vi "Initialize Serial Arm.vi"   [LabVIEW 2017, in "NI_Robotics_AnalyticKinematics.lvlib"]
doc: "Sets the properties of a serial robot arm and generates a representation of the arm. If you have access to a 6R, 5R, or SCARA arm, generate that type of arm. If you do not have access to an arm of those types, generate a generic arm. You must manually select the polymorphic instance to use."
uses:
  <vilib>/robotics/Kinematics/Analytical/NI_Robotics_AnalyticKinematics.lvlib
  <vilib>/robotics/Kinematics/Analytical/6R/Type 1/NI_Robotics_6R Type 1 Serial Arm Class.lvclass
  <vilib>/robotics/Kinematics/Robot/NI_Robotics_Serial Robot Arm.lvclass
  <vilib>/robotics/Kinematics/Analytical/SCARA/NI_Robotics_SCARA Serial Arm Class.lvclass
  <vilib>/robotics/Kinematics/Analytical/6R/Type 3/NI_Robotics_6R Type 3 Serial Arm Class.lvclass
  <vilib>/robotics/Kinematics/Analytical/6R/Type 2/NI_Robotics_6R Type 2 Serial Arm Class.lvclass
  <vilib>/robotics/Kinematics/Analytical/5R/Type 1/NI_Robotics_5R Type 1 Serial Arm Class.lvclass
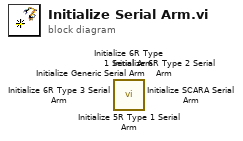
[diagram p0: block diagram]
diagram:
  n1 = call <vilib>:"Initialize 5R Type 1 Serial Arm.vi"() -> ()  [unwired: 10 in, 2 out]
  n2 = call <vilib>:"Initialize 6R Type 2 Serial Arm.vi"() -> ()  [unwired: 10 in, 2 out]
  n3 = call <vilib>:"Initialize 6R Type 3 Serial Arm.vi"() -> ()  [unwired: 10 in, 2 out]
  n4 = call <vilib>:"Initialize SCARA Serial Arm.vi"() -> ()  [unwired: 10 in, 2 out]
  n5 = call <vilib>:"Initialize Generic Serial Arm.vi"() -> ()  [unwired: 10 in, 2 out]
  n6 = call <vilib>:"Initialize 6R Type 1 Serial Arm.vi"() -> ()  [unwired: 10 in, 2 out]
